vi "pressure_main.vi"(8 "Error In":errorcluster, 11 "main_FGV_data":T1={"pipe_properties"={"out_radius"=0.0, "in_radius"=0.0, "out_diameter"=0.0, "in_diameter"=0.0, "thickness"=0.0, "inertia"=0.0, "area"=0.0}, "DirPath"=path "L:/Documentos/00 SERVIÇOS/Tensão residual/Olapa 10-2017/Dados/Primeira Seção/Furos", "DirReport"=path "L:/Documentos/00 SERVIÇOS/Tensão residual/Olapa 10-2017/RelatóriosOlapa/Teste", "Points"=[], "ovalization_data"={"AngOval"=[0.0, 60.0, 120.0, 22.5, 45.0, 67.5, 90.0, 112.5, 135.0, 157.5, 180.0], "OvalDiam"=[324.25, 324.6, 324.55, 324.25, 324.55, 324.65, 324.6, 324.65, 324.55, 324.5, 324.4], "Plots"={"Ref"={"X"=[], "Y"=[]}, "Elipse"={"X"=[], "Y"=[]}, "Points"={"X"=[], "Y"=[]}}, "Ampliation"=100.0, "Results"={"MD"=0.0, "mD"=0.0, "Dmed"=0.0, "Oval"=0.0, "ang"=0.0, "X0"=0.0, "Y0"=0.0}}, "StressDist_data"={"Long"={"Plot"=[], "Fit"=[], "ColorMap"=[], "Data"=[], "peirce_data"={"Plot"=[], "Index removidos"=[]}}, "Circ"={"Plot"=[], "Fit"=[], "ColorMap"=[], "Data"=[], "peirce_data"={"Plot"=[], "Index removidos"=[]}}, "Shear"={"Plot"=[], "Fit"=[], "ColorMap"=[], "Data"=[], "peirce_data"={"Plot"=[], "Index removidos"=[]}}, "Equivalent"={"Plot"=[], "Fit"=[], "ColorMap"=[], "Data"=[], "peirce_data"={"Plot"=[], "Index removidos"=[]}}}, "pressure_data"={"Pressure"=[], "StressCircOval"=[], "StressCirc"=[], "StressLong"=[], "Plot"=[], "Angle"=[]}}) -> (0 "Error Out":errorcluster, 3 "main_FGV_data-out":T1={"pipe_properties"={"out_radius"=0.0, "in_radius"=0.0, "out_diameter"=0.0, "in_diameter"=0.0, "thickness"=0.0, "inertia"=0.0, "area"=0.0}, "DirPath"=path "L:/Documentos/00 SERVIÇOS/Tensão residual/Olapa 10-2017/Dados/Primeira Seção/Furos", "DirReport"=path "L:/Documentos/00 SERVIÇOS/Tensão residual/Olapa 10-2017/RelatóriosOlapa/Teste", "Points"=[], "ovalization_data"={"AngOval"=[0.0, 60.0, 120.0, 22.5, 45.0, 67.5, 90.0, 112.5, 135.0, 157.5, 180.0], "OvalDiam"=[324.25, 324.6, 324.55, 324.25, 324.55, 324.65, 324.6, 324.65, 324.55, 324.5, 324.4], "Plots"={"Ref"={"X"=[], "Y"=[]}, "Elipse"={"X"=[], "Y"=[]}, "Points"={"X"=[], "Y"=[]}}, "Ampliation"=100.0, "Results"={"MD"=0.0, "mD"=0.0, "Dmed"=0.0, "Oval"=0.0, "ang"=0.0, "X0"=0.0, "Y0"=0.0}}, "StressDist_data"={"Long"={"Plot"=[], "Fit"=[], "ColorMap"=[], "Data"=[], "peirce_data"={"Plot"=[], "Index removidos"=[]}}, "Circ"={"Plot"=[], "Fit"=[], "ColorMap"=[], "Data"=[], "peirce_data"={"Plot"=[], "Index removidos"=[]}}, "Shear"={"Plot"=[], "Fit"=[], "ColorMap"=[], "Data"=[], "peirce_data"={"Plot"=[], "Index removidos"=[]}}, "Equivalent"={"Plot"=[], "Fit"=[], "ColorMap"=[], "Data"=[], "peirce_data"={"Plot"=[], "Index removidos"=[]}}}, "pressure_data"={"Pressure"=[], "StressCircOval"=[], "StressCirc"=[], "StressLong"=[], "Plot"=[], "Angle"=[]}})   [LabVIEW 2016]
uses:
  MainFGV/main_FGV_data.ctl
  MainFGV/pipe_properties.ctl
  StressCalculations/point_data.ctl
  Ovalization/ovalization_data.ctl
  StressDist/StressDist_data.ctl
  StressDist/StressDist_single_data.ctl
  StressDist/Peirce/peirce_data.ctl
  pressure_data.ctl
  <vilib>/Analysis/1siggen.llb/Ramp Pattern by Samples.vi
  <vilib>/Analysis/baseanly.llb/Mean (DBL).vi
  <vilib>/Analysis/NI_AALBase.lvlib
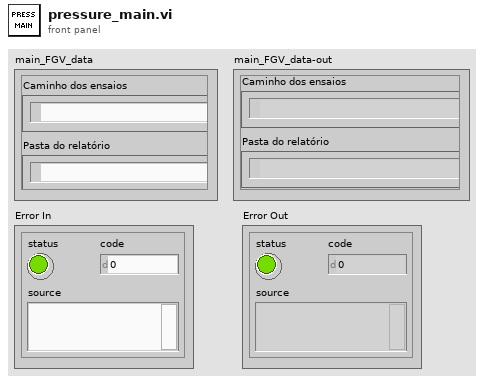
[diagram p1: front panel]
types:
  T1 = typedef "main_FGV_data.ctl" = cluster{"pipe_properties":T2, "DirPath":path, "DirReport":path, "Points":T3[], "ovalization_data":T4, "StressDist_data":T5, "pressure_data":T8}
  T2 = typedef "pipe_properties.ctl" = cluster{"out_radius":dbl, "in_radius":dbl, "out_diameter":dbl, "in_diameter":dbl, "thickness":dbl, "inertia":dbl, "area":dbl}
  T3 = typedef "point_data.ctl" = cluster{"LongStress":dbl, "CircStress":dbl, "ShearStress":dbl, "Pressure":dbl, "Angle":dbl, "Thickness":dbl, "HoleDiam":dbl, "EquiStress":dbl, "S1":dbl, "S2":dbl, "Beta":dbl}
  T4 = typedef "ovalization_data.ctl" = cluster{"AngOval":dbl[], "OvalDiam":dbl[], "Plots":cluster{"Ref":cluster{"X":dbl[], "Y":dbl[]}, "Elipse":cluster{"X":dbl[], "Y":dbl[]}, "Points":cluster{"X":dbl[], "Y":dbl[]}}, "Ampliation":dbl, "Results":cluster{"MD":dbl, "mD":dbl, "Dmed":dbl, "Oval":dbl, "ang":dbl, "X0":dbl, "Y0":dbl}}
  T5 = typedef "StressDist_data.ctl" = cluster{"Long":T6, "Circ":T6, "Shear":T6, "Equivalent":T6}
  T6 = typedef "StressDist_single_data.ctl" = cluster{"Plot":cluster{"Angle":dbl[], "Stress":dbl[]}[], "Fit":dbl[], "ColorMap":dbl[][], "Data":string[][], "peirce_data":T7}
  T7 = typedef "peirce_data.ctl" = cluster{"Plot":cluster{"Array":dbl[], "Array":dbl[]}[], "Index removidos":i32[]}
  T8 = typedef "pressure_data.ctl" = cluster{"Pressure":dbl[], "StressCircOval":dbl[], "StressCirc":dbl[], "StressLong":dbl[], "Plot":cluster{"Angle":dbl[], "Stress":dbl[]}[], "Angle":dbl[]}
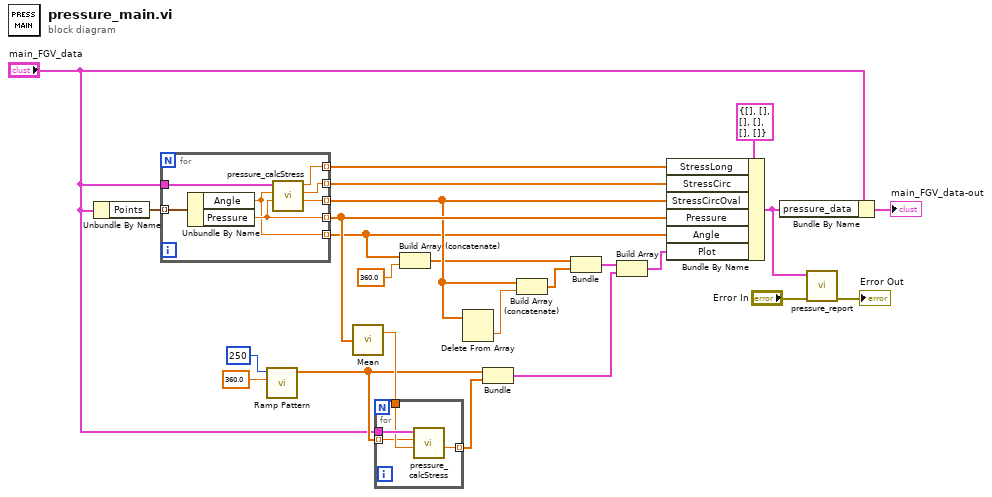
[diagram p0: block diagram]
diagram:
  n1 = Unbundle By Name("main_FGV_data") -> ("Points"=w23:T3[])
  n2 = for {
    tunnel: "main_FGV_data" -> [w31]
    tunnel: w23 -> [w30] mode=indexing
    tunnel: [w29] -> w22 mode=indexing
    tunnel: [w28] -> w21 mode=indexing
    tunnel: [w27] -> w13 mode=indexing
    tunnel: [w26] -> w18 mode=indexing
    tunnel: [w25] -> w4 mode=indexing
    n3 = Unbundle By Name(w30) -> ("Angle"=w25:dbl, "Pressure"=w26:dbl)
    n4 = call "pressure_calcStress.vi"("Pressure"=w26, "Angle"=w25, "main_FGV_data"=w31) -> ("PressCircOval"=w27:dbl, "PressCirc"=w28:dbl, "PressLong"=w29:dbl)  [unwired: 6 in]
  }
  n5 = call-poly <vilib>:"Ramp Pattern.vi"("end"=360.0, "samples"=250) -> ("Ramp Pattern"=w15:dbl[])  [unwired: 8 in, 1 out]
  n6 = call-poly <vilib>:"Mean.vi"("X"=w18) -> ("mean"=w17:dbl)  [unwired: 1 out]
  n7 = for {
    tunnel: "main_FGV_data" -> [w35]
    tunnel: [w34] -> w16 mode=indexing
    tunnel: w17 -> [w33]
    tunnel: w15 -> [w32] mode=indexing
    n8 = call "pressure_calcStress.vi"("Pressure"=w33, "Angle"=w32, "main_FGV_data"=w35) -> ("PressCircOval"=w34:dbl)  [unwired: 6 in, 2 out]
  }
  n9 = Build Array (concatenate)(w4, 360.0) -> (w11:dbl[])
  n10 = Delete From Array(array=w13) -> (deleted portion=w12:dbl)  [unwired: 2 in, 1 out]
  n11 = Bundle("Ramp Pattern"=w15, w16) -> (w8:cluster{"Ramp Pattern":dbl[], dbl[]})  [unwired: 1 in]
  n12 = Build Array (concatenate)(w13, w12) -> (w10:dbl[])
  n13 = Bundle(w11, w10) -> (w9:cluster{dbl[], dbl[]})  [unwired: 1 in]
  n14 = Build Array(w9, w8) -> (w7:cluster{"Ramp Pattern":dbl[], dbl[]}[])
  n15 = Bundle By Name(cluster=T8 {"Pressure"=[], "StressCircOval"=[], "StressCirc"=[], "StressLong"=[], "Plot"=[], "Angle"=[]} ("pressure_data"), "StressLong"=w22, "StressCirc"=w21, "StressCircOval"=w13, "Pressure"=w18, "Angle"=w4, "Plot"=w7) -> (w3:T8)
  n16 = Bundle By Name(cluster="main_FGV_data", "pressure_data"=w3) -> (→"main_FGV_data-out":T1)
  n17 = call "pressure_report.vi"("Error In"="Error In", "Pressure data"=w3) -> ("Error Out"=→"Error Out":errorcluster)  [unwired: 9 in]
